vi "insert-cmd-to-dev.vi"(9 "字符串":string, 10 "枚举":T2(ring), 11 "dev-cmd":T1) -> (3 "dev-cmd out":T1)   [LabVIEW 2019]
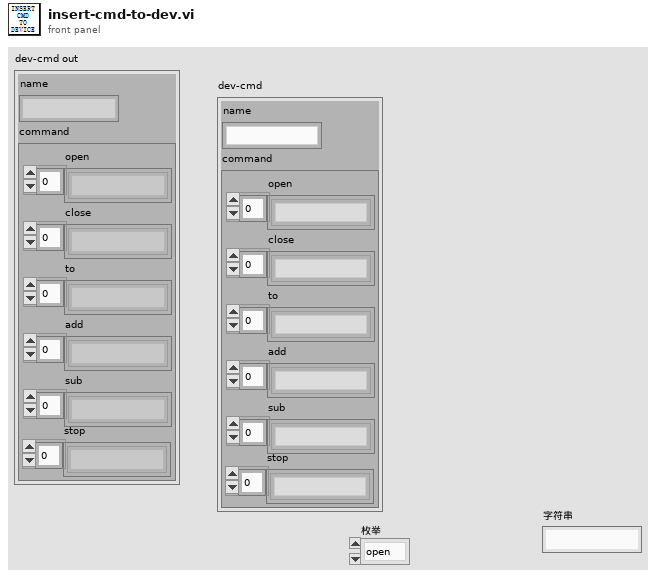
[diagram p1: front panel]
types:
  T1 = cluster{"command":cluster{"open":string[], "close":string[], "to":string[], "add":string[], "sub":string[], "stop":string[]}, "name":string}
  T2 = enum16{"open", "close", "to", "add", "sub", "stop"}
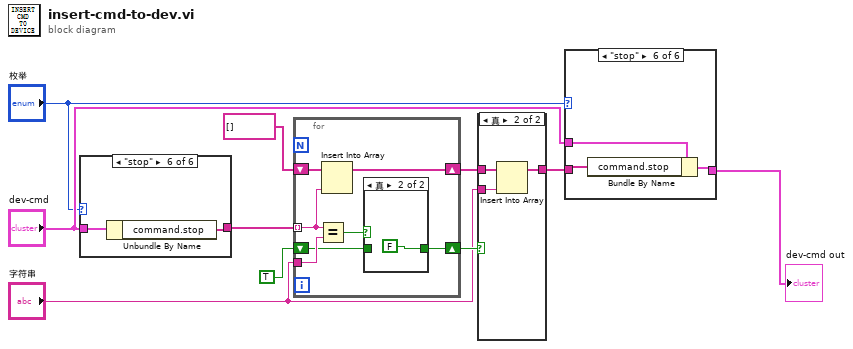
[diagram p0: block diagram]
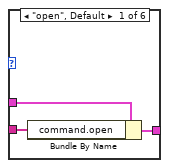
[diagram p2: hidden frame]
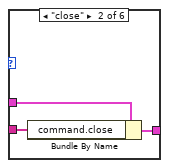
[diagram p3: hidden frame]
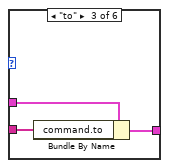
[diagram p4: hidden frame]
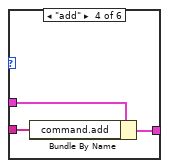
[diagram p5: hidden frame]
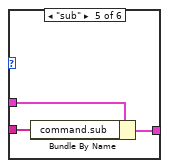
[diagram p6: hidden frame]
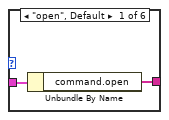
[diagram p9: hidden frame]
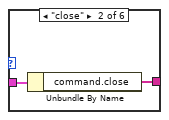
[diagram p10: hidden frame]
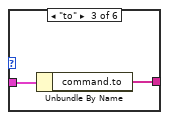
[diagram p11: hidden frame]
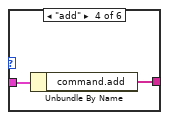
[diagram p12: hidden frame]
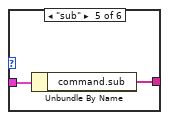
[diagram p13: hidden frame]
diagram:
  n1 = case shown="\"stop\"" "枚举" {
    tunnel: "dev-cmd" -> [w11 w14 w16 w18 w20 w22]
    tunnel: [w12 w13 w15 w17 w19 w21] -> w10
    frame "open", Default {
      n2 = Unbundle By Name(w11) -> ("command.open"=w12:string[])
    }
    frame "close" {
      n3 = Unbundle By Name(w14) -> ("command.close"=w13:string[])
    }
    frame "to" {
      n4 = Unbundle By Name(w16) -> ("command.to"=w15:string[])
    }
    frame "add" {
      n5 = Unbundle By Name(w18) -> ("command.add"=w17:string[])
    }
    frame "sub" {
      n6 = Unbundle By Name(w20) -> ("command.sub"=w19:string[])
    }
    frame "stop" {
      n7 = Unbundle By Name(w22) -> ("command.stop"=w21:string[])
    }
  }
  n8 = for {
    tunnel: w10 -> [w25] mode=indexing
    tunnel: "字符串" -> [w29]
    shift-right: [w27] -> w7
    shift-left: TRUE ("x = y?") -> [w26]
    shift-right: [w23] -> w6
    shift-left: string[] [] -> [w24]
    n9 = Equal?(x=w25, y=w29) -> (x = y?=w28:bool)
    n10 = Insert Into Array(array=w24, new element=w25) -> (w23:string[])  [unwired: 1 in]
    n11 = case shown="真" w28 {
      tunnel: [w30 FALSE ("x = y?")] -> w27
      tunnel: w26 -> [w30 _]
      frame False {
      }
      frame True {
      }
    }
  }
  n12 = case shown="真" w7 {
    tunnel: w6 -> [w32 w35]
    tunnel: "字符串" -> [_ w34]
    tunnel: [w32 w33] -> w3
    frame False {
    }
    frame True {
      n13 = Insert Into Array(array=w35, new element=w34) -> (w33:string[])  [unwired: 1 in]
    }
  }
  n14 = case shown="\"stop\"" "枚举" {
    tunnel: "dev-cmd" -> [w38 w41 w43 w46 w50 w51]
    tunnel: w3 -> [w37 w39 w42 w45 w48 w52]
    tunnel: [w36 w40 w44 w47 w49 w53] -> w1
    frame "open", Default {
      n15 = Bundle By Name(cluster=w38, "command.open"=w37) -> (w36:T1)
    }
    frame "close" {
      n16 = Bundle By Name(cluster=w41, "command.close"=w39) -> (w40:T1)
    }
    frame "to" {
      n17 = Bundle By Name(cluster=w43, "command.to"=w42) -> (w44:T1)
    }
    frame "add" {
      n18 = Bundle By Name(cluster=w46, "command.add"=w45) -> (w47:T1)
    }
    frame "sub" {
      n19 = Bundle By Name(cluster=w50, "command.sub"=w48) -> (w49:T1)
    }
    frame "stop" {
      n20 = Bundle By Name(cluster=w51, "command.stop"=w52) -> (w53:T1)
    }
  }
  "dev-cmd out" <- w1
